vi "global-JKISMQ FGV Change Flag.vi"() -> ()   [LabVIEW 2014, in "JKI-State-Machine-Plus.lvlib"]
uses:
  JKI-State-Machine-Plus.lvlib
panel:
  in  "global-JKISMQ FGV Change Flag":u32
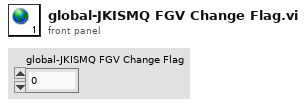
[diagram p1: front panel]
diagram:
